vi "Write to TimeTest DB_Test VI.vi"() -> ()   [LabVIEW 2014]
uses:
  ftw-dataflow/ftw/src/core/time/FTW-Time-DisplayFormat-Timestamp.ctl
  <vilib>/addons/database/Connection.llb/DB Tools Open Connec (Path).vi
  <vilib>/addons/database/NI_Database_API.lvlib
panel:
  out "data":string[][](table)
  out "date/time string":string
  out "Formatted Timestamp":string
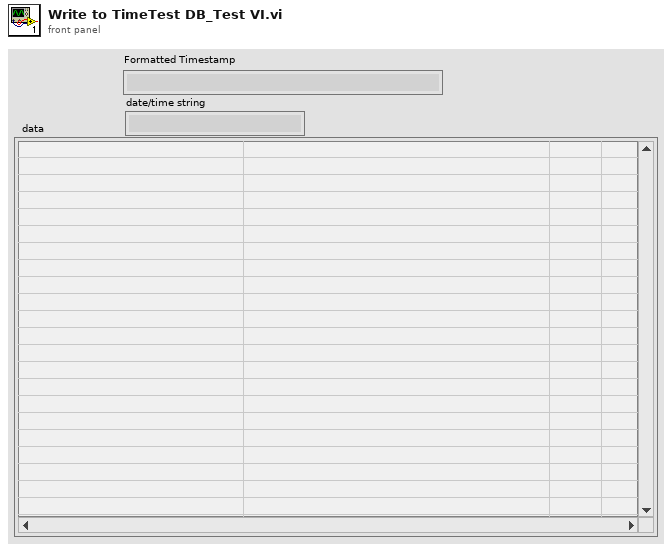
[diagram p1: front panel]
types:
  T1 = typedef "FTW-Time-DisplayFormat-Timestamp.ctl" = enum16{"YYYY-MM-DDT00:00:00.000Z (ISO-8601)", "YYYY-MM-DDT00-00-00Z (Simple ISO-8601)", "YYYY-MM-DD"}
  T2 = typedef "NI_Database_API.lvlib/Conn ObjectReference.ctl" = refnum<k1>
  T3 = cluster{"Formatted Timestamp":string, "date/time string":string}
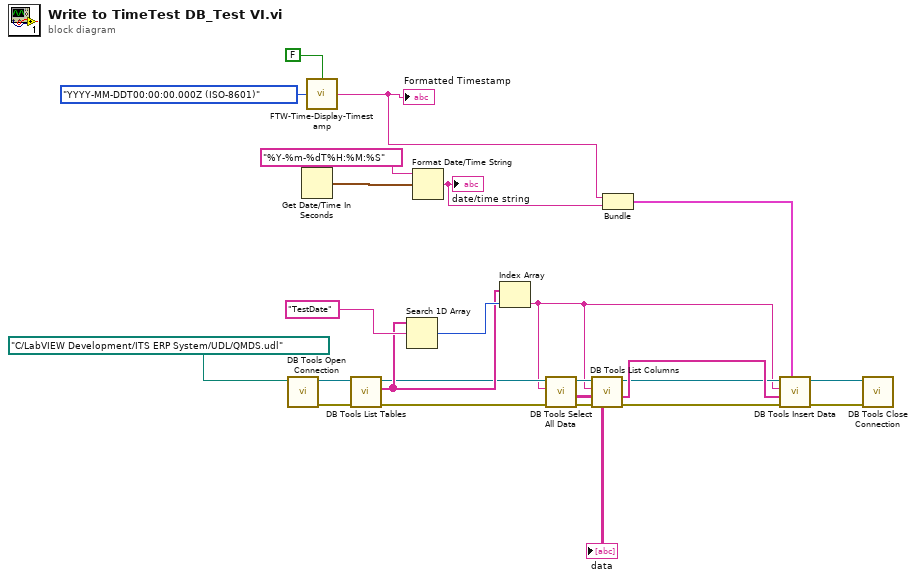
[diagram p0: block diagram]
diagram:
  n1 = call-poly <vilib>:"DB Tools Open Connection.vi"("connection information"=path "C:/LabVIEW Development/ITS ERP System/UDL/QMDS.udl" ("Database (mdb)  File Path")) -> ("error out"=w11:errorcluster, "connection reference"=w12:T2)  [unwired: 7 in]
  n2 = Get Date/Time In Seconds() -> (seconds since 1Jan1904=w2:timestamp)
  n3 = call "FTW-Time-Display-Timestamp.vi"("Zulu?"=FALSE, "Format"=FTW-Time-DisplayFormat-Timestamp."YYYY-MM-DDT00:00:00.000Z (ISO-8601)") -> ("Formatted Timestamp"=w1:string)  [unwired: 2 in]
  "Formatted Timestamp" <- w1
  n4 = call <vilib>:"DB Tools List Tables.vi"("error in (no error)"=w11, "connection reference"=w12) -> ("error out"=w17:errorcluster, "tables"=w21:string[], "connection reference out"=w19:T2)  [unwired: 3 in]
  n5 = Search 1D Array(1D array=w21, element="TestDate" ("Table")) -> (index of element=w23:i32)  [unwired: 1 in]
  n6 = Format Date/Time String(time format string (%c)="%Y-%m-%dT%H:%M:%S", seconds (now)=w2) -> (date/time string=w6:string)  [unwired: 1 in]
  "date/time string" <- w6
  n7 = Index Array(array=w21, index=w23) -> (element=w13:string)
  n8 = call <vilib>:"DB Tools Select All Data.vi"("error in (no error)"=w17, "table"=w13, "connection reference"=w19) -> ("error out"=w18:errorcluster, "data"=→"data":string[][], "connection reference out"=w20:T2)  [unwired: 3 in]
  n9 = call <vilib>:"DB Tools List Columns.vi"("error in (no error)"=w18, "table"=w13, "connection reference"=w20) -> ("error out"=w16:errorcluster, "columns"=w15:string[], "connection reference out"=w14:T2)  [unwired: 1 in, 1 out]
  n10 = Bundle("Formatted Timestamp"=w1, "date/time string"=w6) -> (w10:T3)  [unwired: 1 in]
  n11 = call <vilib>:"DB Tools Insert Data.vi"("data"=w10, "error in (no error)"=w16, "columns"=w15, "table"=w13, "connection reference"=w14) -> ("error out"=w8:errorcluster, "connection reference out"=w9:T2)  [unwired: 5 in]
  n12 = call <vilib>:"DB Tools Close Connection.vi"("error in (no error)"=w8, "connection reference"=w9) -> ()  [unwired: 5 in, 1 out]
